vi "Launch New Service.vi"(8 "error in (no error)":errorcluster, 10 "Service Type":T1, 11 "Manager in":refnum<class "Manager.lvclass">) -> (0 "error out":errorcluster, 3 "Manager out":refnum<class "Manager.lvclass">)   [LabVIEW 2016, in "Manager.lvlib" / "Manager.lvclass"]
uses:
  Manager.lvclass
  C:/Program Files (x86)/National Instruments/LabVIEW 2016/vi.lib/ActorFramework/Actor/Actor.lvclass
  Service Types.ctl
  Client/Client/Client.lvclass
  Manager.lvclass/Manager.ctl
  Client/Client/Client.lvclass/Client.ctl
  Server/Server/Server.lvclass
  <vilib>/ActorFramework/Actor/Actor.lvclass
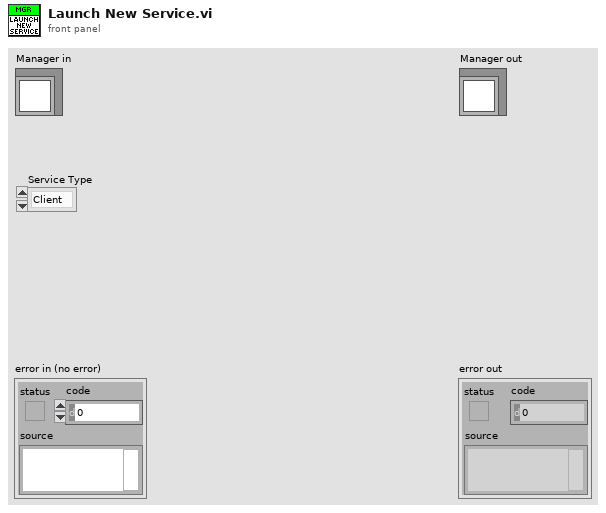
[diagram p1: front panel]
types:
  T1 = typedef "Manager.lvlib/Manager.lvclass/Service Types.ctl" = enum16{"Client", "Server"}
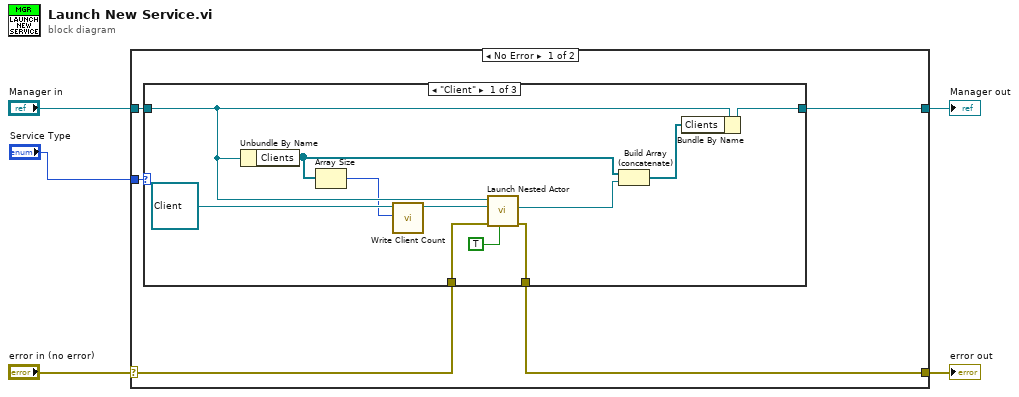
[diagram p0: block diagram]
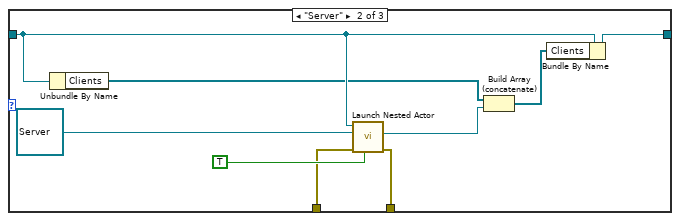
[diagram p2: hidden frame]
diagram:
  n1 = case shown="No Error" "error in (no error)" {
    selector: "error in (no error)" -> [w10 w34]
    tunnel: [w9 w34] -> w4
    tunnel: [w7 w33] -> w2
    tunnel: "Manager in" -> [w8 w33]
    tunnel: "Service Type" -> [w6 _]
    frame No Error {
      n2 = case shown="\"Client\"" w6 {
        tunnel: w10 -> [w19 w28 w31]
        tunnel: [w18 w27 w31] -> w9
        tunnel: w8 -> [w17 w26 w32]
        tunnel: [w15 w23 w32] -> w7
        frame "Client" {
          n3 = Unbundle By Name(w17) -> ("Clients"=w12:refnum<class "Message Enqueuer.lvclass">[])
          n4 = Array Size(array=w12) -> (size(s)=w11:i32)
          n5 = call "Write Client Count.vi"("Client Count"=w11, "Client in"=refnum<class "Client.lvclass"> refnum ("Client.lvlib:Client.lvclass")) -> ("Client out"=w13:refnum<class "Client.lvclass">)  [unwired: 9 in]
          n6 = call <vilib>:"Launch Nested Actor.vi"("Open Actor Core front panel? (F)"=TRUE, "error in (no error)"=w19, "Nested Actor"=w13, "Caller Actor in"=w17) -> ("error out"=w18:errorcluster, "Nested Actor's Enqueuer"=w16:refnum<class "Message Enqueuer.lvclass">)  [unwired: 5 in, 1 out]
          n7 = Build Array (concatenate)(w12, w16) -> (w14:refnum<class "Message Enqueuer.lvclass">[])
          n8 = Bundle By Name(cluster=w17, "Clients"=w14) -> (w15:refnum<class "Manager.lvclass">)
        }
        frame "Server" {
          n9 = Unbundle By Name(w26) -> ("Clients"=w25:refnum<class "Message Enqueuer.lvclass">[])
          n10 = call <vilib>:"Launch Nested Actor.vi"("Open Actor Core front panel? (F)"=TRUE, "error in (no error)"=w28, "Nested Actor"=refnum<class "Server.lvclass"> refnum ("Server.lvlib:Server.lvclass"), "Caller Actor in"=w26) -> ("error out"=w27:errorcluster, "Nested Actor's Enqueuer"=w24:refnum<class "Message Enqueuer.lvclass">)  [unwired: 5 in, 1 out]
          n11 = Build Array (concatenate)(w25, w24) -> (w22:refnum<class "Message Enqueuer.lvclass">[])
          n12 = Bundle By Name(cluster=w26, "Clients"=w22) -> (w23:refnum<class "Manager.lvclass">)
        }
        frame Default {
        }
      }
    }
    frame Error {
    }
  }
  "error out" <- w4
  "Manager out" <- w2
